vi "Display Setup.vi"(0 "VISA resource name":refnum<visa-resource-name>, 5 "Enable Display (T: Enable)":bool=TRUE, 7 "Display Mode (0: Normal)":u16(ring) items=["Normal", "Text"], 9 "Text Input":string, 11 "error in (no error)":errorcluster) -> (4 "VISA resource name out":refnum<visa-resource-name>, 15 "error out":errorcluster)   [LabVIEW 2021, in "Agilent 34420.lvlib"]
doc: "Configures the display settings of the instrument."
uses:
  <instrlib>/Agilent 34420/Agilent 34420.lvlib
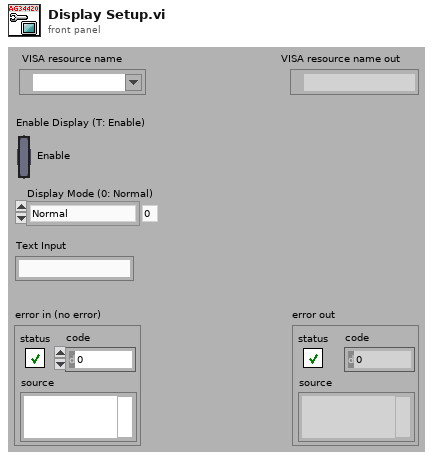
[diagram p1: front panel]
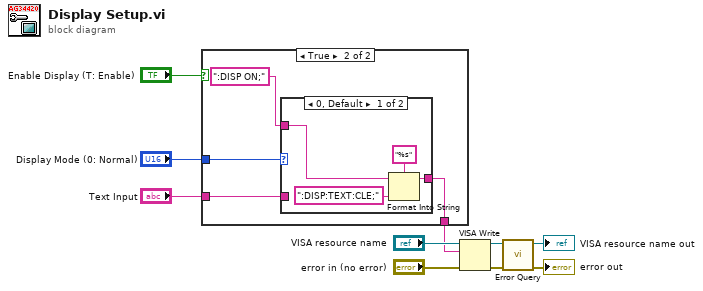
[diagram p0: block diagram]
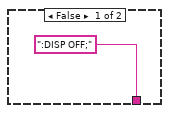
[diagram p2: hidden frame]
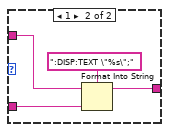
[diagram p3: hidden frame]
diagram:
  n1 = case shown="True" "Enable Display (T: Enable)" {
    tunnel: "Display Mode (0: Normal)" -> [_ w15]
    tunnel: [":DISP OFF;" ("output string") w12] -> w2
    tunnel: "Text Input" -> [_ w13]
    frame False {
    }
    frame True {
      n2 = case shown="0, Default" w15 {
        tunnel: ":DISP ON;" -> [w18 w21]
        tunnel: w13 -> [_ w23]
        tunnel: [w16 w20] -> w12
        frame 0, Default {
          n3 = Format Into String(format string="%s", initial string=w18, ":DISP:TEXT:CLE;") -> (resulting string=w16:string)  [unwired: 1 in, 1 out]
        }
        frame 1 {
          n4 = Format Into String(format string=":DISP:TEXT \"%s\";", initial string=w21, w23) -> (resulting string=w20:string)  [unwired: 1 in, 1 out]
        }
      }
    }
  }
  n5 = VISA Write(VISA resource name="VISA resource name", write buffer=w2, error in (no error)="error in (no error)") -> (VISA resource name out=w6:refnum<visa-resource-name>, error out=w5:errorcluster)  [unwired: 1 out]
  n6 = call <instrlib>:"Error Query.vi"("error in (no error)"=w5, "VISA resource name"=w6) -> ("error out"=→"error out":errorcluster, "VISA resource name out"=→"VISA resource name out":refnum<visa-resource-name>)  [unwired: 6 in, 2 out]
